vi "Convert Raw to HEX.vi"(4 "Raw Data Flattened to String":string) -> (1 "Hex String":string)   [LabVIEW 2017]
doc: "Converts Raw Data that has been flattened to a string into ASCII HEX (printable characters with no control codes)"
panel:
  out "length":i32
  out "Hex Data":i32[](array[numeric]) format="%x"
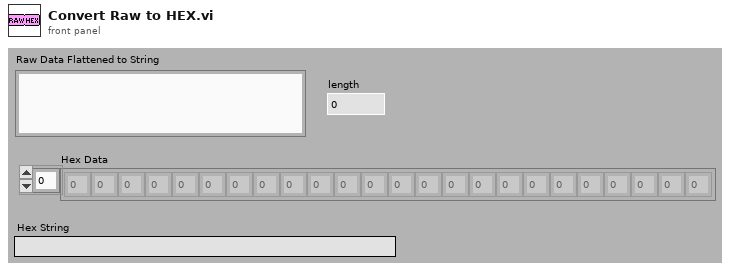
[diagram p1: front panel]
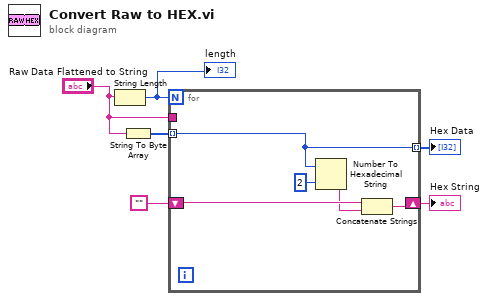
[diagram p0: block diagram]
diagram:
  n1 = String Length(string="Raw Data Flattened to String") -> (length=w6:i32)
  "length" <- w6
  n2 = String To Byte Array(string="Raw Data Flattened to String") -> (unsigned byte array=w1:u8[])
  n3 = for {
    N: w6 -> [_]
    tunnel: [w7] -> w5 mode=indexing
    tunnel: "Raw Data Flattened to String" -> [_]
    shift-right: [w9] -> w3
    shift-left: "" -> [w11]
    tunnel: w1 -> [w7] mode=indexing
    n4 = Number To Hexadecimal String(1:i16 2 ("width (-)"), 2:w7) -> (0:w10:string)
    n5 = Concatenate Strings(w11, w10) -> (w9:string)
  }
  "Hex Data" <- w5
  "Hex String" <- w3
